vi "Write Module Slot.vi"(6 "Module Slot":T1={"Slot State"=enum."Empty", "BBM Type"=enum."BBM", "HDI Type"=enum."HDI", "Vacuum Channel"=0, "Location/Orientation BBM"={"Center"=refnum, "Orientation"=refnum}, "Location/Orientation HDI"={"Center"=refnum, "Orientation"=refnum}, "S/N"=""}, 8 "error in":errorcluster, 9 "slot":i32, 10 "chuck":i32, 11 "WorkTable in":refnum<class "WorkTable Class.lvclass">) -> (0 "error out":errorcluster, 3 "WorkTable out":refnum<class "WorkTable Class.lvclass">)   [LabVIEW 2011, in "WorkTable Class.lvclass"]
uses:
  WorkTable Class.lvclass
  Type Definitions/Worktable_Module Slot.ctl
  Vec3d Class/Vec3d Class.lvclass
  Orient3d Class/Orient3d Class.lvclass
  Utils/Type Definitions/Position_Orientation.ctl
  WorkTable Class.lvclass/WorkTable Class.ctl
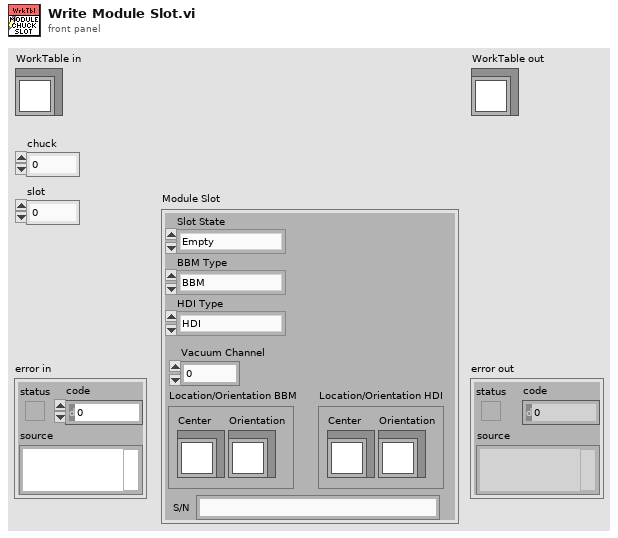
[diagram p1: front panel]
types:
  T1 = typedef "Worktable_Module Slot.ctl" = cluster{"Slot State":enum16{"Empty", "Unglued", "Stamped", "PartOnTop", "Weighted", "Unpotted", "Potted"}, "BBM Type":enum16{"None", "BBM", "GlassSlide"}, "HDI Type":enum16{"None", "HDI", "Polyimide"}, "Vacuum Channel":u8, "Location/Orientation BBM":T2, "Location/Orientation HDI":T2, "S/N":string}
  T2 = typedef "Position_Orientation.ctl" = cluster{"Center":refnum<class "Vec3d Class.lvclass">, "Orientation":refnum<class "Orient3d Class.lvclass">}
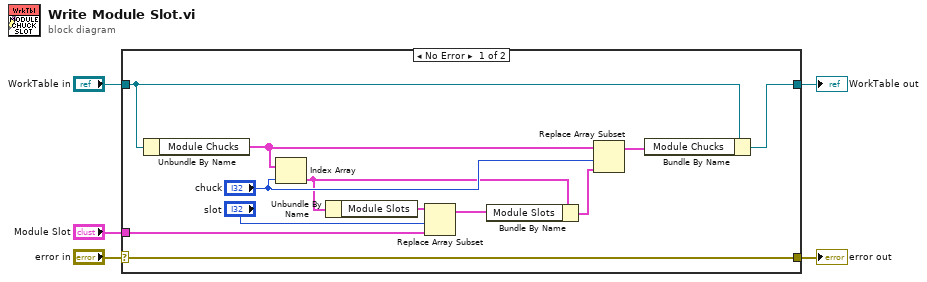
[diagram p0: block diagram]
diagram:
  n1 = case shown="No Error" "error in" {
    selector: "error in" -> [w17 w18]
    tunnel: [w17 w18] -> w4
    tunnel: [w16 w19] -> w2
    tunnel: "WorkTable in" -> [w15 w19]
    tunnel: "Module Slot" -> [w12 _]
    frame No Error {
      n2 = Unbundle By Name(w15) -> ("Module Chucks"=w11:cluster{"Module Slots":T1[]}[])
      n3 = Index Array(array=w11, index="chuck") -> (element=w9:cluster{"Module Slots":T1[]})
      n4 = Unbundle By Name(w9) -> ("Module Slots"=w14:T1[])
      n5 = Replace Array Subset(array=w14, new element=w12, index="slot") -> (w8:T1[])
      n6 = Bundle By Name(cluster=w9, "Module Slots"=w8) -> (w7:cluster{"Module Slots":T1[]})
      n7 = Replace Array Subset(array=w11, new element=w7, index="chuck") -> (w6:cluster{"Module Slots":T1[]}[])
      n8 = Bundle By Name(cluster=w15, "Module Chucks"=w6) -> (w16:refnum<class "WorkTable Class.lvclass">)
    }
    frame Error {
    }
  }
  "error out" <- w4
  "WorkTable out" <- w2
